vi "UI_Configurate.vi"(8 "error in (no error)":errorcluster, 11 "UI_Move.lvclass":refnum<class "UI_Move.lvclass">) -> (0 "error out":errorcluster, 3 "UI_Move.lvclass Out":refnum<class "UI_Move.lvclass">)   [LabVIEW 2015, in "UI_Move.lvclass"]
uses:
  UI_Move.lvclass
  Private/UI_Move Console.vi
panel:
  in  "Pane":refnum<vi>
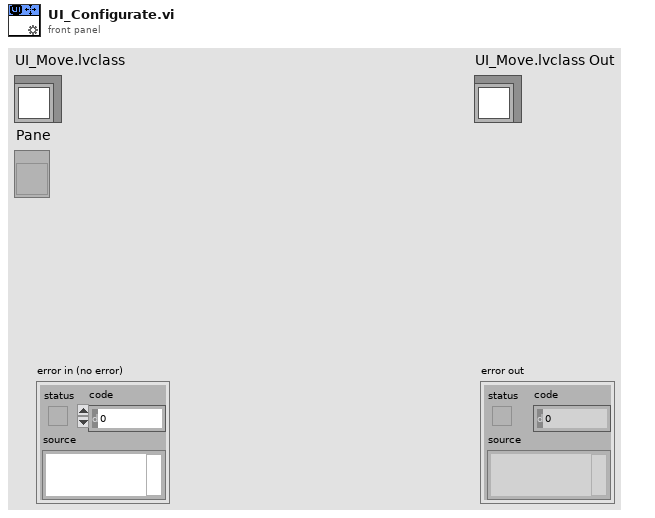
[diagram p1: front panel]
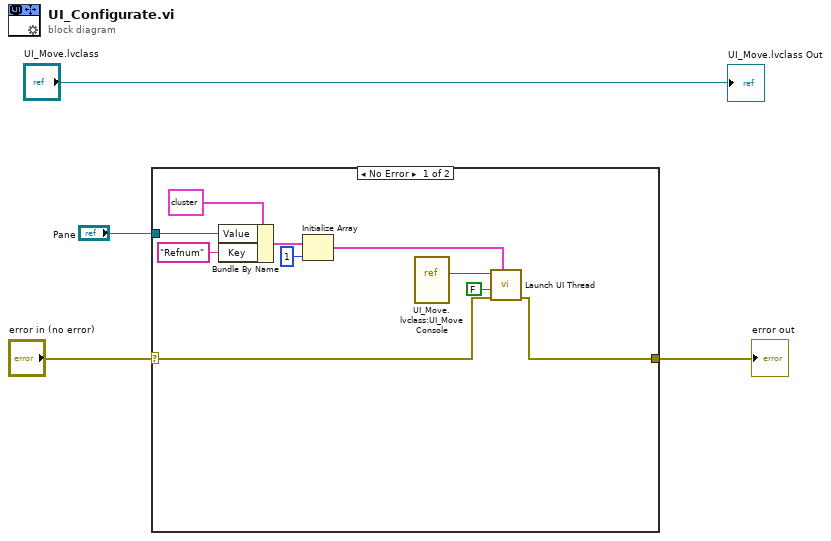
[diagram p0: block diagram]
diagram:
  n1 = case shown="No Error" "error in (no error)" {
    selector: "error in (no error)" -> [w12 w15]
    tunnel: [w11 w15] -> w2
    tunnel: "Pane" -> [w9 _]
    frame No Error {
      n2 = Bundle By Name(cluster=cluster{"Value":variant, "Key":string} {"Value"=variant, "Key"=""}, "Value"=w9, "Key"="Refnum") -> (w7:cluster{"Value":variant, "Key":string})
      n3 = Initialize Array(w7, 1 ("dimension size")) -> (w5:cluster{"Value":variant, "Key":string}[])
      n4 = vi-ref "UI_Move.lvclass:UI_Move Console.vi"() -> (w14:refnum<vi>)
      n5 = call "Launch UI Thread.vi"("VI Extern Value"=w5, "error in (no error)"=w12, "Open?(True)"=FALSE, "This VI"=w14) -> ("error out"=w11:errorcluster)  [unwired: 6 in, 1 out]
    }
    frame Error {
    }
  }
  "error out" <- w2
  "UI_Move.lvclass Out" <- "UI_Move.lvclass"
